vi "process_storage.vi"(6 "error in (no error)":errorcluster) -> (0 "error out":errorcluster)   [LabVIEW 2010]
uses:
  typedefs/control_storage_enum.ctl
  typedefs/data_cluster.ctl
  typedefs/storage_parameters_cluster.ctl
  typedefs/main_state_enum.ctl
panel:
  out "Storing":bool
  out "Current file":path
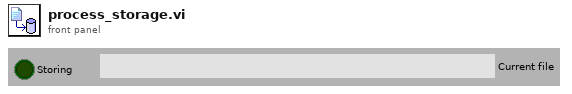
[diagram p1: front panel]
types:
  T1 = typedef "data_cluster.ctl" = cluster{"t0":dbl, "dt":dbl, "Channels":dbl[][]}
  T2 = typedef "control_storage_enum.ctl" = enum16{"Init", "Discard", "Store", "Reset", "Stop", "Quit"}
  T3 = cluster{"Control storage enum":T2, "variant":variant}
  T4 = typedef "storage_parameters_cluster.ctl" = cluster{"Store?":bool, "Path":path, "Basename":string, "Auto-increment?":bool}
  T5 = enum16{"open", "replace", "create", "open or create", "replace or create", "replace or create with confirmation"}
  T6 = typedef "main_state_enum.ctl" = enum16{"Init", "Empty", "ParamsChanged", "Start", "Stop", "Abort", "Acquisition finished", "SetShutter", "Reset", "Error", "Quit"}
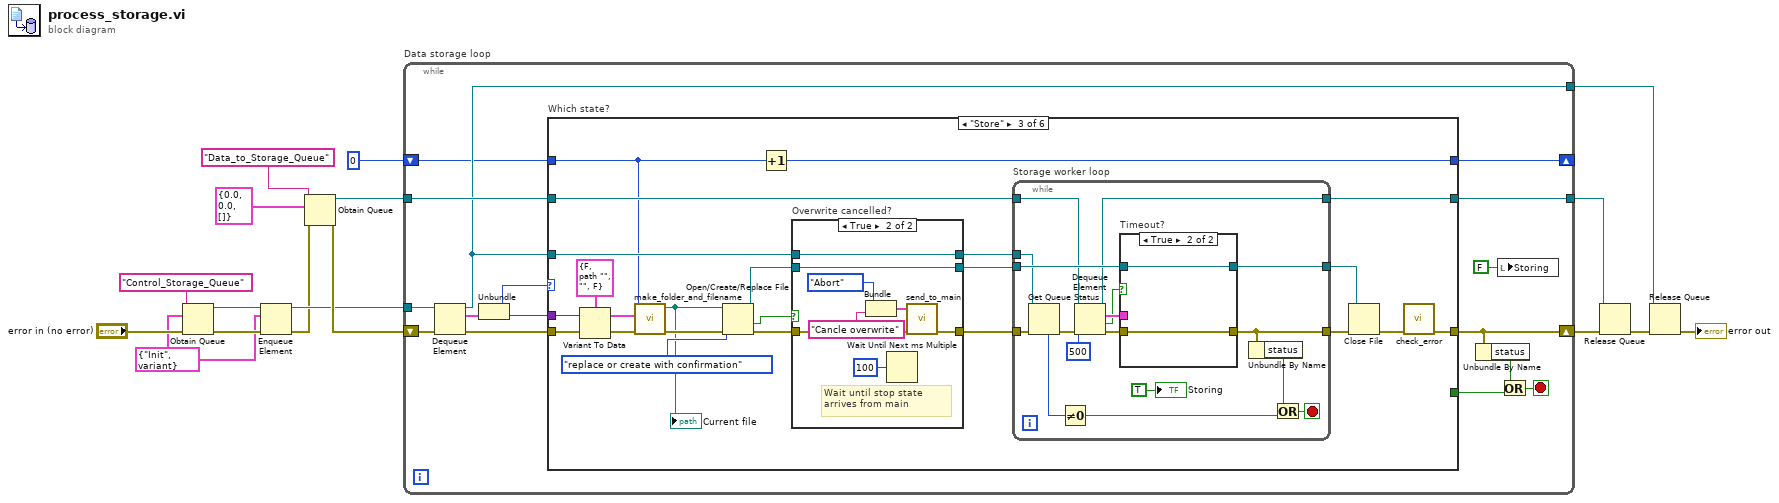
[diagram p0: block diagram]
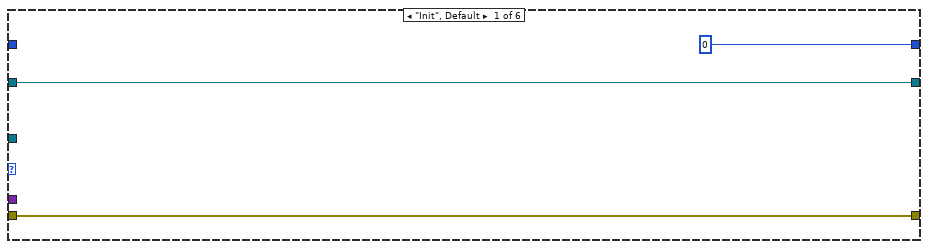
[diagram p2: hidden frame]
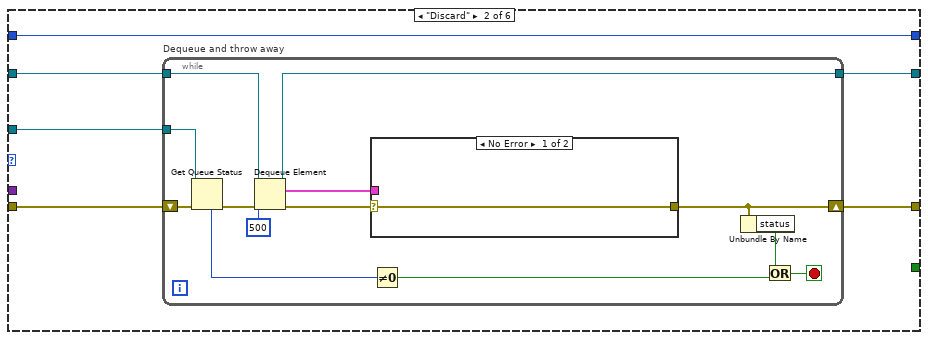
[diagram p3: hidden frame]
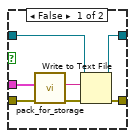
[diagram p6: hidden frame]
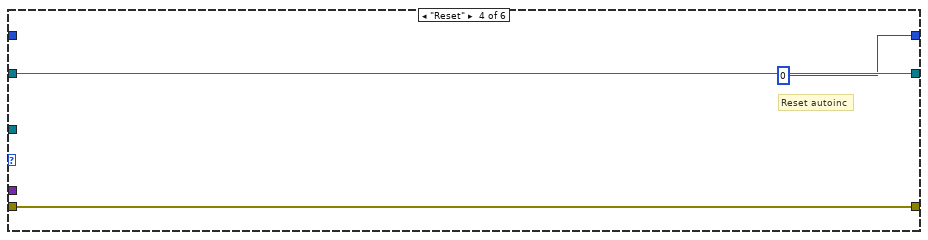
[diagram p7: hidden frame]
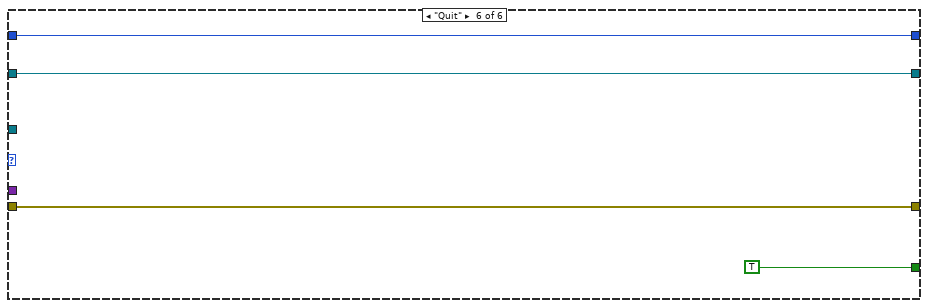
[diagram p9: hidden frame]
diagram:
  w1 = T3 {"Control storage enum"=enum."Init", "variant"=variant}
  n1 = Obtain Queue(name (unnamed)="Control_Storage_Queue", element data type=w1, error in (no error)="error in (no error)") -> (queue out=w5:refnum<queue>, error out=w3:errorcluster)  [unwired: 2 in, 1 out]
  n2 = Enqueue Element(queue=w5, element=w1, error in (no error)=w3) -> (queue out=w4:refnum<queue>, error out=w2:errorcluster)  [unwired: 1 in, 1 out]
  n3 = Obtain Queue(name (unnamed)="Data_to_Storage_Queue", element data type=T1 {"t0"=0.0, "dt"=0.0, "Channels"=[]} ("Data cluster"), error in (no error)=w2) -> (queue out=w9:refnum<queue>, error out=w8:errorcluster)  [unwired: 2 in, 1 out]
  n4 = while "Data storage loop" {
    shift-right: [w25] -> w11
    shift-left: w8 -> [w31]
    tunnel: w4 -> [w32]
    tunnel: [w21] -> w13
    tunnel: w9 -> [w26]
    tunnel: [w33] -> w12
    shift-right: [w19] -> _
    shift-left: 0 ("Fileno.") -> [w20]
    stop <- w23 stop-if-true
    n5 = Dequeue Element(queue=w32, error in (no error)=w31) -> (queue out=w21:refnum<queue>, element=w30:T3, error out=w27:errorcluster)  [unwired: 1 in, 1 out]
    n6 = Unbundle(w30) -> ("Control storage enum"=w29:T2, "variant"=w28:variant)
    n7 = case "Which state?" shown="\"Store\"" w29 {
      tunnel: [w36 w39 w77 w120 w123 w127] -> w33
      tunnel: w28 -> [_ _ w79 _ _ _]
      tunnel: w27 -> [w34 w40 w80 w119 w122 w125]
      tunnel: w26 -> [w36 w42 w78 w120 w123 w127]
      tunnel: [w34 w38 w70 w119 w122 w125] -> w25
      tunnel: [_ _ _ _ _ TRUE] -> w22
      tunnel: w21 -> [_ w41 w64 _ _ _]
      tunnel: w20 -> [_ w37 w60 _ w121 w124]
      tunnel: [0 ("Fileno.") w37 w72 0 ("Fileno.") w121 w124] -> w19
      frame "Init", Default {
      }
      frame "Discard" {
        n8 = while "Dequeue and throw away" {
          tunnel: w42 -> [w49]
          tunnel: w41 -> [w54]
          shift-right: [w44] -> w38
          shift-left: w40 -> [w55]
          tunnel: [w46] -> w39
          stop <- w51 stop-if-true
          n9 = Get Queue Status(queue=w54, error in (no error)=w55) -> (error out=w50:errorcluster, # elements in queue=w53:i32)  [unwired: 1 in, 6 out]
          n10 = Dequeue Element(queue=w49, timeout in ms (-1)=500, error in (no error)=w50) -> (queue out=w46:refnum<queue>, element=w43:T1, error out=w45:errorcluster)  [unwired: 1 out]
          n11 = case shown="No Error" w45 {
            selector: w45 -> [w56 w57]
            tunnel: [w56 w57] -> w44
            tunnel: w43 -> [_ _]
            frame No Error {
            }
            frame Error {
            }
          }
          n12 = Not Equal To 0?(x=w53) -> (x != 0?=w52:bool)
          n13 = Unbundle By Name(w44) -> ("status"=w47:bool)
          n14 = Or(x=w47, y=w52) -> (x .or. y?=w51:bool)
        }
      }
      frame "Store" {
        n15 = Variant To Data(error in=w80, Variant=w79, type=T4 {"Store?"=FALSE, "Path"=path "", "Basename"="", "Auto-increment?"=FALSE} ("Storage parameters")) -> (error out=w62:errorcluster, data=w59:T4)
        n16 = call "make_folder_and_filename.vi"("error in (no error)"=w62, "Storage parameters"=w59, "Fileno"=w60) -> ("error out"=w61:errorcluster, "Path"=w58:path)  [unwired: 7 in]
        "Current file" <- w58
        n17 = Open/Create/Replace File(file path (use dialog)=w58, error in=w61, operation (0:open)=T5."replace or create with confirmation") -> (refnum out=w66:refnum<file>, cancelled=w67:bool, error out=w69:errorcluster)  [unwired: 3 in]
        n18 = Increment(x=w60) -> (x+1=w72:i32)
        n19 = case "Overwrite cancelled?" shown="True" w67 {
          tunnel: w69 -> [w83 w88]
          tunnel: [w83 w87] -> w68
          tunnel: w66 -> [w82 w91]
          tunnel: [w82 w91] -> w65
          tunnel: [w81 w90] -> w63
          tunnel: w64 -> [w81 w90]
          frame False {
          }
          frame True {
            # "Wait until stop state arrives from main"
            n20 = Bundle("State Enum"=main_state_enum."Abort", "Cancle overwrite") -> (w86:cluster{"State Enum":T6, string})  [unwired: 1 in]
            n21 = Wait Until Next ms Multiple(millisecond multiple=u32 100) -> ()  [unwired: 1 out]
            n22 = call "send_to_main.vi"("error in (no error)"=w88, "Main state cluster"=w86) -> ("error out"=w87:errorcluster)  [unwired: 9 in]
          }
        }
        n23 = while "Storage worker loop" {
          tunnel: w78 -> [w98]
          tunnel: [w95] -> w76
          tunnel: w65 -> [w107]
          tunnel: [w106] -> w75
          tunnel: w68 -> [w105]
          tunnel: w63 -> [w103]
          tunnel: [w97] -> w77
          stop <- w99 stop-if-true
          n24 = Get Queue Status(queue=w103, error in (no error)=w105) -> (error out=w104:errorcluster, # elements in queue=w101:i32)  [unwired: 1 in, 6 out]
          n25 = Not Equal To 0?(x=w101) -> (x != 0?=w100:bool)
          n26 = Dequeue Element(queue=w98, timeout in ms (-1)=500, error in (no error)=w104) -> (queue out=w97:refnum<queue>, element=w108:T1, timed out?=w93:bool, error out=w92:errorcluster)
          n27 = case "Timeout?" shown="True" w93 {
            tunnel: [w115 w116] -> w95
            tunnel: w108 -> [w110 _]
            tunnel: w107 -> [w113 w117]
            tunnel: [w114 w117] -> w106
            tunnel: w92 -> [w109 w116]
            frame False {
              n28 = call "pack_for_storage.vi"("error in"=w109, "Data in"=w110) -> ("error out"=w112:errorcluster, "String out"=w111:string)  [unwired: 8 in]
              n29 = Write to Text File(file (use dialog)=w113, text=w111, error in=w112) -> (refnum out=w114:refnum<file>, error out=w115:errorcluster)  [unwired: 1 in, 1 out]
            }
            frame True {
            }
          }
          n30 = Unbundle By Name(w95) -> ("status"=w102:bool)
          n31 = Or(x=w102, y=w100) -> (x .or. y?=w99:bool)
          "Storing" <- TRUE ("Storing")
        }
        n32 = Close File(refnum=w75, error in=w76) -> (error out=w71:errorcluster)  [unwired: 1 out]
        n33 = call "check_error.vi"("error in"=w71) -> ("error out"=w70:errorcluster)  [unwired: 10 in]
      }
      frame "Reset" {
        # "Reset autoinc"
      }
      frame "Stop" {
      }
      frame "Quit" {
      }
    }
    n34 = Unbundle By Name(w25) -> ("status"=w24:bool)
    n35 = local write "Storing"(FALSE ("Storing")) -> ()
    n36 = Or(x=w24, y=w22) -> (x .or. y?=w23:bool)
  }
  n37 = Release Queue(queue=w12, error in (no error)=w11) -> (error out=w10:errorcluster)  [unwired: 1 in, 2 out]
  n38 = Release Queue(queue=w13, error in (no error)=w10) -> (error out=→"error out":errorcluster)  [unwired: 1 in, 2 out]
